vi "Export_Update Device.vi"(11 "Export Setting in":T1) -> (3 "Export Setting out":T1)   [LabVIEW 2015, in "ConfigHelper.lvlib"]
uses:
  ConfigHelper.lvlib
  Control_UI_Export Setting.ctl
  Control_UI_Export Setting State.ctl
  <vilib>/addons/PointValueMap/controls/PointMap.ctl
  Control_Export File Setup.ctl
  <vilib>/addons/PointValueMap/PointValueMap.lvlib
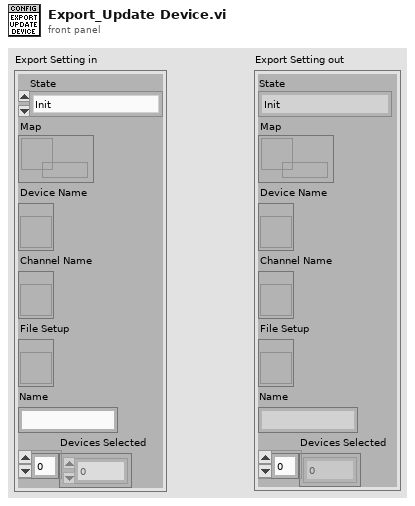
[diagram p1: front panel]
types:
  T1 = typedef "ConfigHelper.lvlib/Control_UI_Export Setting.ctl" = cluster{"State":T2, "Map":T3, "Device Name":refnum<vi>, "Channel Name":refnum<vi>, "File Setup":refnum<vi>, "Name":string, "Devices Selected":i32[]}
  T2 = typedef "ConfigHelper.lvlib/Control_UI_Export Setting State.ctl" = enum16{"Init", "Wait", "Exit", "Write to File", "Read from PVM", "Write to PVM", "Update Device", "Add Device", "Remove Device", "Copy Device", "Update Channel", "Add Channel", "Remove Channel", "Import from TDMS"}
  T3 = typedef "PointValueMap.lvlib/PointMap.ctl" = refnum<data-value>
  T4 = enum8{"Enabled", "Disabled", "Disabled and Grayed Out"}
  T5 = typedef "ConfigHelper.lvlib/Control_Export File Setup.ctl" = cluster{"CSV":bool, "TDMS":bool, "RAW TDMS":bool}
  T6 = typedef "ConfigHelper.lvlib/Control_Export Setup.ctl" = cluster{"Device Name":string, "Export CSV":bool, "Export TDMS":bool, "Export RAW TDMS":bool, "Channel Names":string[]}
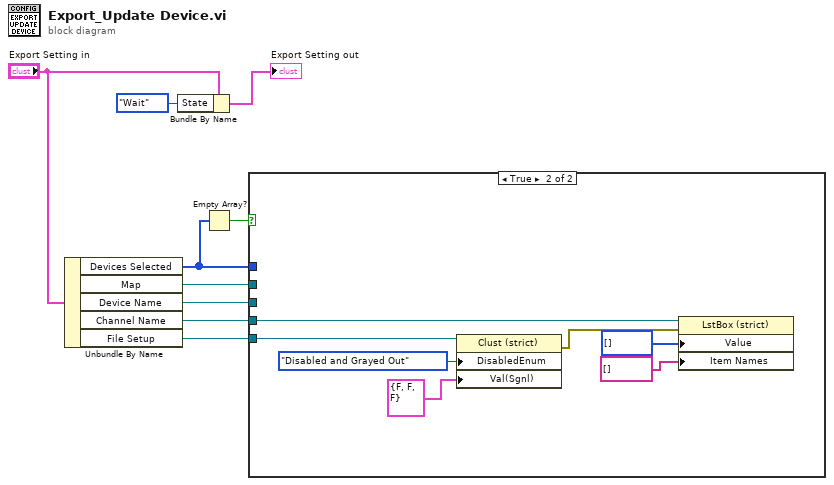
[diagram p0: block diagram]
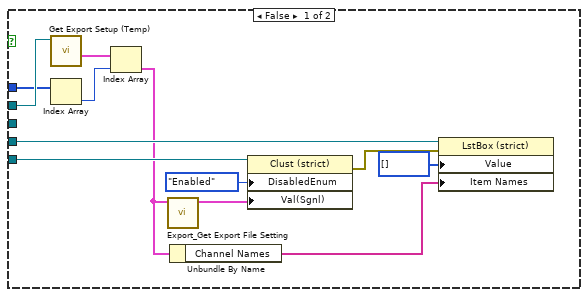
[diagram p2: hidden frame]
diagram:
  n1 = Unbundle By Name("Export Setting in") -> ("Devices Selected"=w1:i32[], "Map"=w5:T3, "Device Name"=w4:refnum<vi>, "Channel Name"=w3:refnum<vi>, "File Setup"=w2:refnum<vi>)
  n2 = Bundle By Name(cluster="Export Setting in", "State"=Control_UI_Export_Setting_State."Wait") -> (→"Export Setting out":T1)
  n3 = Empty Array?(array=w1) -> (empty?=w6:bool)
  n4 = case shown="True" w6 {
    tunnel: w5 -> [w21 _]
    tunnel: w4 -> [_ _]
    tunnel: w3 -> [w14 w25]
    tunnel: w2 -> [w17 w28]
    tunnel: w1 -> [w20 _]
    frame False {
      n5 = call "Get Export Setup (Temp).vi"("Map"=w21) -> ("Export Setup"=w19:T6[])  [unwired: 8 in, 2 out]
      n6 = Index Array(array=w20) -> (element=w18:i32)  [unwired: 1 in]
      n7 = Index Array(array=w19, index=w18) -> (element=w11:T6)
      n8 = call "Export_Get Export File Setting.vi"("Device Export Setup"=w11) -> ("Export File Setting"=w15:T5)  [unwired: 10 in]
      n9 = Unbundle By Name(w11) -> ("Channel Names"=w10:string[])
      n10 = property class="Clust (strict)"(reference=w17, "DisabledEnum"=T4."Enabled" ("Disabled"), "Val(Sgnl)"=w15) -> (error out=w13:errorcluster)  [unwired: 1 in, 1 out]
      n11 = property class="LstBox (strict)"(reference=w14, error in=w13, "Value"=i32[] [], "Item Names"=w10) -> ()  [unwired: 2 out]
    }
    frame True {
      n12 = property class="Clust (strict)"(reference=w28, "DisabledEnum"=T4."Disabled and Grayed Out" ("Disabled"), "Val(Sgnl)"=T5 {"CSV"=FALSE, "TDMS"=FALSE, "RAW TDMS"=FALSE} ("Export File Setup")) -> (error out=w24:errorcluster)  [unwired: 1 in, 1 out]
      n13 = property class="LstBox (strict)"(reference=w25, error in=w24, "Value"=i32[] [], "Item Names"=string[] []) -> ()  [unwired: 2 out]
    }
  }
